vi "test_Tx Exec Unit.vi"() -> ()   [LabVIEW 2020]
uses:
  Engine/Implementation/Tx Execution Unit/Tx Generic Execution Unit.lvclass
  Engine/Interfaces/Shared Resources/Shared Resources.lvclass
  <instrlib>/AIM GmbH/_AIM 664/_controls/queue_header_generic.ctl
  <instrlib>/AIM GmbH/_AIM 664/AIM664LV.lvlib
  Engine/Implementation/Tx Execution Unit/RawFrame.ctl
  Engine/Implementation/Tx Execution Unit/channel_settings_tx.ctl
  Engine/Implementation/Tx Execution Unit/hardware_channels_tx.ctl
  Frame Configuration/controls/frame_record_type.ctl
panel:
  out "Frames":T1[](array[typedef]) {"Data" format="%.0x"; "HeaderInfo"."NetSelect" items=["FDX_TX_FRAME_DLY_A"=0, "FDX_TX_FRAME_DLY_B"=1, "FDX_TX_FRAME_BOTH "=3, "FDX_TX_FRAME_ONLY_A"=4, "FDX_TX_FRAME_ONLY_B "=5]; "HeaderInfo"."FrameStartMode" items=["FDX_TX_FRAME_START_IFG", "FDX_TX_FRAME_START_PGWT", "FDX_TX_FRAME_START_TRG"]; "HeaderInfo"."PhysErrorInjection" items=["FDX_TX_FRAME_ERR_OFF"=0, "FDX_TX_FRAME_ERR_CRC"=1, "FDX_TX_FRAME_ERR_ALI"=2, "FDX_TX_FRAME_ERR_PRE"=4, "FDX_TX_FRAME_ERR_PHY"=8]; "HeaderInfo"."SequenceNumberInit" items=["FDX_TX_FRAME_SEQ_INIT_AUTO"=65535]; "HeaderInfo"."SequenceNumberOffset" items=["FDX_TX_FRAME_SEQ_OFFS_AUTO "=65535]; "HeaderInfo"."PayloadGenerationMode" items=["FDX_TX_FRAME_PGM_USER"=0, "FDX_TX_FRAME_PGM_IP_PART"=1, "FDX_TX_FRAME_PGM_IP_FULL"=2, "FDX_TX_FRAME_PGM_IP_PART_TT"=10, "FDX_TX_FRAME_PGM_IP_FULL_TT"=20]; "HeaderInfo"."PayloadBufferMode" items=["FDX_TX_FRAME_PBM_STD", "FDX_TX_FRAME_PBM_MAC", "FDX_TX_FRAME_PBM_UDP"]}
  in  "file path (use dialog)":path=path "/home/admin/1Frame_10mS.bin"
  out "Values out":dbl[](array[numeric])
  in  "TX Parameters":T3={"channel #"=0, "channel handle"=0, "InstrumentHandle_board"=0, "InstrumentHandle_port"=0, "channel settings"={"Tx Board"=0, "Tx Port"=0, "Frame Array"=[], "QueueSizeIn"=1}} {"channel settings"."Frame Array"."Data" format="%.0x"; "channel settings"."Frame Array"."HeaderInfo"."NetSelect" items=["FDX_TX_FRAME_DLY_A"=0, "FDX_TX_FRAME_DLY_B"=1, "FDX_TX_FRAME_BOTH "=3, "FDX_TX_FRAME_ONLY_A"=4, "FDX_TX_FRAME_ONLY_B "=5]; "channel settings"."Frame Array"."HeaderInfo"."FrameStartMode" items=["FDX_TX_FRAME_START_IFG", "FDX_TX_FRAME_START_PGWT", "FDX_TX_FRAME_START_TRG"]; "channel settings"."Frame Array"."HeaderInfo"."PhysErrorInjection" items=["FDX_TX_FRAME_ERR_OFF"=0, "FDX_TX_FRAME_ERR_CRC"=1, "FDX_TX_FRAME_ERR_ALI"=2, "FDX_TX_FRAME_ERR_PRE"=4, "FDX_TX_FRAME_ERR_PHY"=8]; "channel settings"."Frame Array"."HeaderInfo"."SequenceNumberInit" items=["FDX_TX_FRAME_SEQ_INIT_AUTO"=65535]; "channel settings"."Frame Array"."HeaderInfo"."SequenceNumberOffset" items=["FDX_TX_FRAME_SEQ_OFFS_AUTO "=65535]; "channel settings"."Frame Array"."HeaderInfo"."PayloadGenerationMode" items=["FDX_TX_FRAME_PGM_USER"=0, "FDX_TX_FRAME_PGM_IP_PART"=1, "FDX_TX_FRAME_PGM_IP_FULL"=2, "FDX_TX_FRAME_PGM_IP_PART_TT"=10, "FDX_TX_FRAME_PGM_IP_FULL_TT"=20]; "channel settings"."Frame Array"."HeaderInfo"."PayloadBufferMode" items=["FDX_TX_FRAME_PBM_STD", "FDX_TX_FRAME_PBM_MAC", "FDX_TX_FRAME_PBM_UDP"]}
  out "error out":errorcluster
  in  "stop":bool
  in  "loop rate mS":u32=10
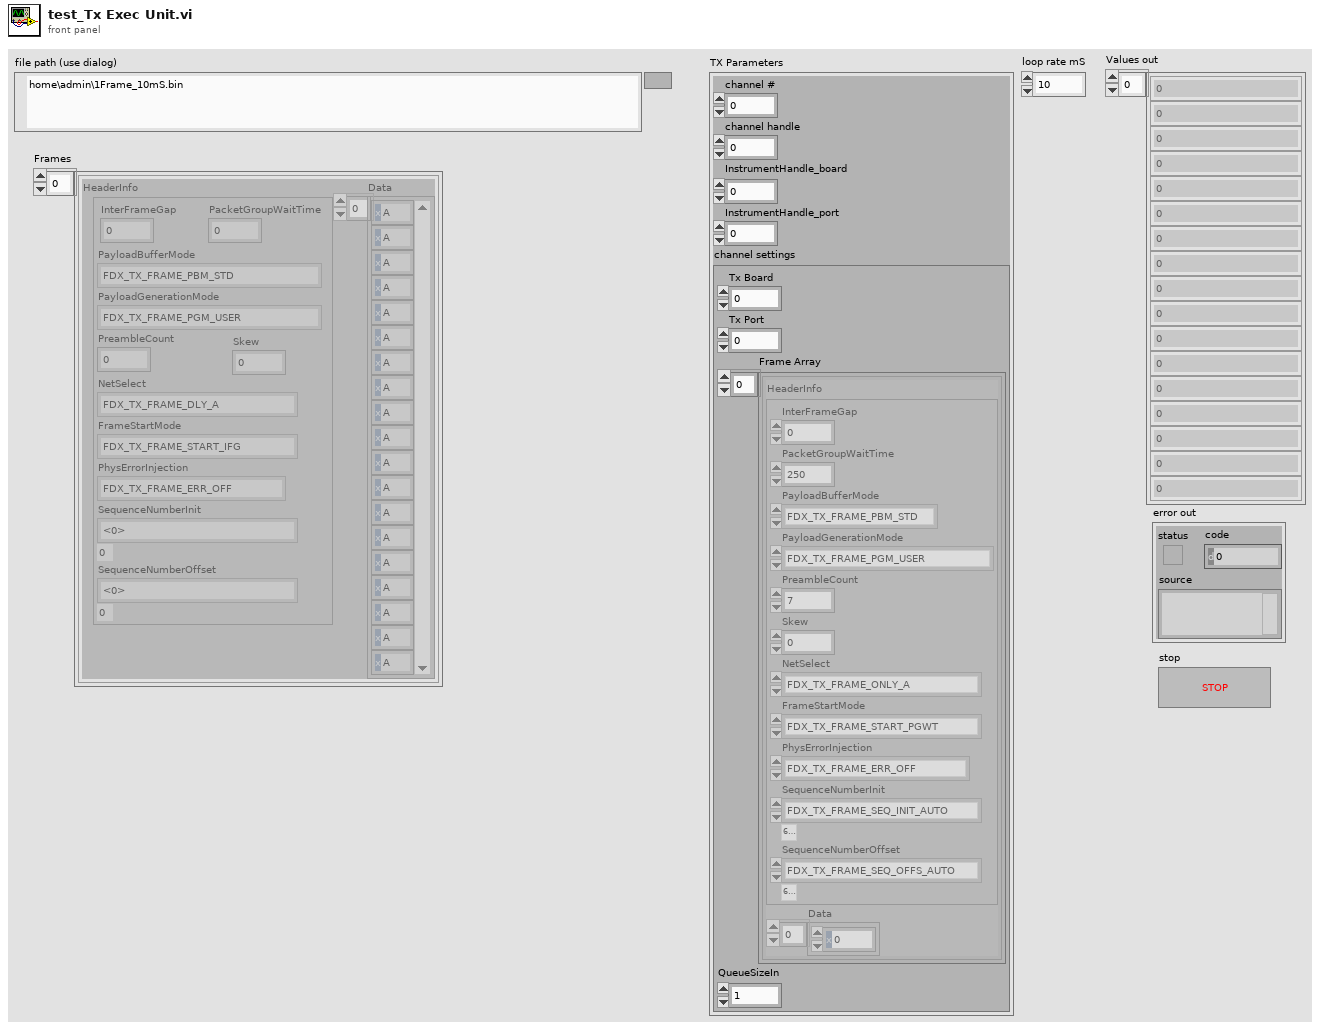
[diagram p1: front panel]
types:
  T1 = typedef "frame_record_type.ctl" = cluster{"HeaderInfo":T2, "Data":u8[]}
  T2 = typedef "AIM664LV.lvlib/queue_header_generic.ctl" = cluster{"InterFrameGap":u32, "PacketGroupWaitTime":u32, "PayloadBufferMode":u8, "PayloadGenerationMode":u8, "PreambleCount":u8, "Skew":u32, "NetSelect":u8, "FrameStartMode":u8, "PhysErrorInjection":u32, "SequenceNumberInit":u16, "SequenceNumberOffset":u16}
  T3 = typedef "AIM ARINC 664 Engine.lvlib/Implementation.lvlib/Tx Generic Execution Unit.lvclass/hardware_channels_tx.ctl" = cluster{"channel #":u16, "channel handle":u64, "InstrumentHandle_board":u32, "InstrumentHandle_port":u32, "channel settings":T4}
  T4 = typedef "AIM ARINC 664 Engine.lvlib/Implementation.lvlib/Tx Generic Execution Unit.lvclass/channel_settings_tx.ctl" = cluster{"Tx Board":u32, "Tx Port":u32, "Frame Array":T5[], "QueueSizeIn":u32}
  T5 = typedef "AIM ARINC 664 Engine.lvlib/Implementation.lvlib/Tx Generic Execution Unit.lvclass/RawFrame.ctl" = cluster{"HeaderInfo":T2, "Data":u8[]}
  T6 = typedef "frame_file_entry.ctl" = cluster{"key":string, "value":T1}
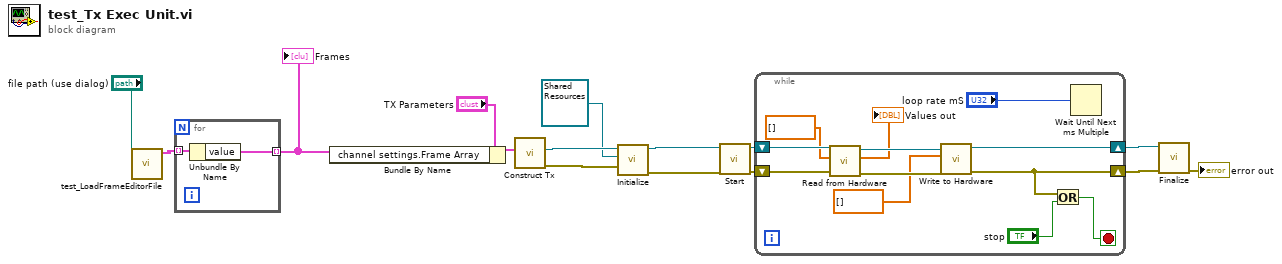
[diagram p0: block diagram]
diagram:
  n1 = call "test_LoadFrameEditorFile.vi"("file path (use dialog)"="file path (use dialog)") -> ("data"=w3:T6[])  [unwired: 9 in, 1 out]
  n2 = for {
    tunnel: w3 -> [w17] mode=indexing
    tunnel: [w16] -> w2 mode=indexing
    n3 = Unbundle By Name(w17) -> ("value"=w16:T1)
  }
  "Frames" <- w2
  n4 = Bundle By Name(cluster="TX Parameters", "channel settings.Frame Array"=w2) -> (w4:T3)
  n5 = call "Construct Tx.vi"("TX Parameters"=w4) -> ("error out"=w7:errorcluster, "Tx Execution Unit out"=w15:refnum<class "Tx Generic Execution Unit.lvclass">)  [unwired: 7 in, 1 out]
  n6 = call-dynamic "Initialize.vi"("error in"=w7, "shared resources"=refnum<class "Shared Resources.lvclass"> refnum, "Tx Execution Unit Implementation in"=w15) -> ("error out"=w9:errorcluster, "Tx Execution Unit Implementation out"=w14:refnum<class "Tx Generic Execution Unit.lvclass">)  [unwired: 7 in]
  n7 = call-dynamic "Start.vi"("error in"=w9, "Tx Execution Unit Implementation in"=w14) -> ("error out"=w12:errorcluster, "Tx Execution Unit Implementation out"=w13:refnum<class "Tx Generic Execution Unit.lvclass">)  [unwired: 8 in]
  n8 = while {
    shift-right: [w25] -> w11
    shift-left: w13 -> [w29]
    shift-right: [w23] -> w10
    shift-left: w12 -> [w28]
    stop <- w21 stop-if-true
    n9 = call-dynamic "Read from Hardware.vi"("error in"=w28, "Values in"=dbl[] [], "Tx Execution Unit Implementation in"=w29) -> ("error out"=w26:errorcluster, "Values out"=→"Values out":dbl[], "Tx Execution Unit Implementation out"=w27:refnum<class "Tx Generic Execution Unit.lvclass">)  [unwired: 6 in]
    n10 = call-dynamic "Write to Hardware.vi"("error in"=w26, "Values in"=dbl[] [], "Tx Execution Unit Implementation in"=w27) -> ("error out"=w23:errorcluster, "Tx Execution Unit Implementation out"=w25:refnum<class "Tx Generic Execution Unit.lvclass">)  [unwired: 5 in, 2 out]
    n11 = Or(x=w23, y="stop") -> (x .or. y?=w21:bool)
    n12 = Wait Until Next ms Multiple(millisecond multiple="loop rate mS") -> ()  [unwired: 1 out]
  }
  n13 = call-dynamic "Finalize.vi"("error in"=w10, "Tx Execution Unit in"=w11) -> ("error out"=→"error out":errorcluster)  [unwired: 8 in, 1 out]
